vi "Set_Rescaling_Setting.vi"(6 "isOriginalMonitor":bool, 8 "error in (no error)":errorcluster, 9 "avg":dbl, 10 "PowerMonitorType":enum16{"DAQ", "MPM_220", "TSL_LOGG"}(ring), 11 ".NET Reference in":refnum<k24>) -> (0 "error out":errorcluster, 3 "Reference out":refnum<k24>)   [LabVIEW 2017]
doc: "Setting for STS rescaling mode"
uses:
  D:/test/ILSTS/LV_IL/LV_IL_Sample_x86/DLL/STSProcess.dll
  DLL/STSProcess.dll
panel:
  in  "mode":i32(ring) items=["Freerun_SPU", "Freerun_Referencemodule"]
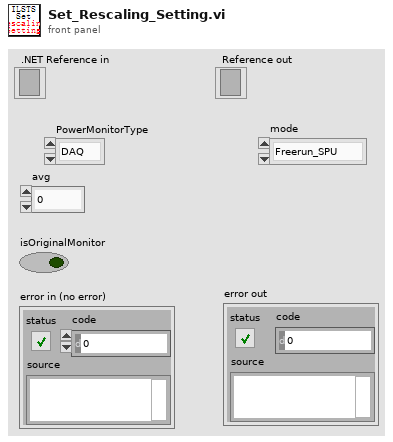
[diagram p1: front panel]
types:
  T1 = enum16{"Freerun_SPU", "Freerun_Referencemodule", "Freerun_TSLMonitor"}
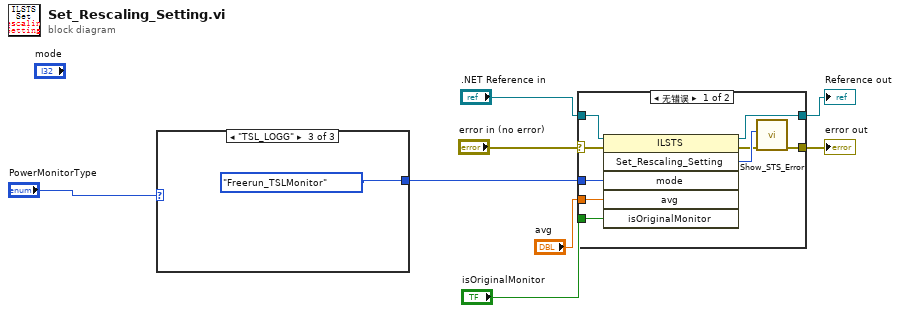
[diagram p0: block diagram]
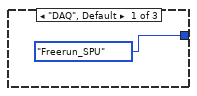
[diagram p2: hidden frame]
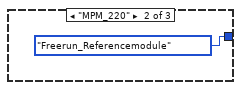
[diagram p3: hidden frame]
diagram:
  n1 = case shown="\"TSL_LOGG\"" "PowerMonitorType" {
    tunnel: [T1."Freerun_SPU" T1."Freerun_Referencemodule" T1."Freerun_TSLMonitor"] -> w1
    frame "DAQ", Default {
    }
    frame "MPM_220" {
    }
    frame "TSL_LOGG" {
    }
  }
  n2 = case shown="无错误" "error in (no error)" {
    selector: "error in (no error)" -> [w18 w22]
    tunnel: ".NET Reference in" -> [w20 w21]
    tunnel: [w19 w21] -> w7
    tunnel: [w15 w22] -> w5
    tunnel: w1 -> [w14 _]
    tunnel: "avg" -> [w13 _]
    tunnel: "isOriginalMonitor" -> [w12 _]
    frame No Error {
      n3 = invoke on="调用节点" class="ILSTS" method="Set_Rescaling_Setting"(reference=w20, error in=w18, "mode"=w14, "avg"=w13, "isOriginalMonitor"=w12) -> (reference out=w19:refnum<k24>, error out=w16:errorcluster, "Set_Rescaling_Setting"=w17:i32)  [unwired: 1 in, 3 out]
      n4 = call "Show_STS_Error.vi"("error in (no error)"=w16, "Error"=w17) -> ("error out"=w15:errorcluster)  [unwired: 9 in]
    }
    frame Error {
    }
  }
  "error out" <- w5
  "Reference out" <- w7
